vi "FTT Init Display.vi"(8 "error in (no error)":errorcluster caption="错误输入（无错误）", 11 "Cluster 2":T4) -> (0 "error out":errorcluster caption="错误输出", 3 "Cluster out":T4)   [LabVIEW 2014]
uses:
  <vilib>/picture/picture.llb/imagedata.ctl
  Type'def/CN Config Ctr.ctl
  Type'def/CN image Ctr.ctl
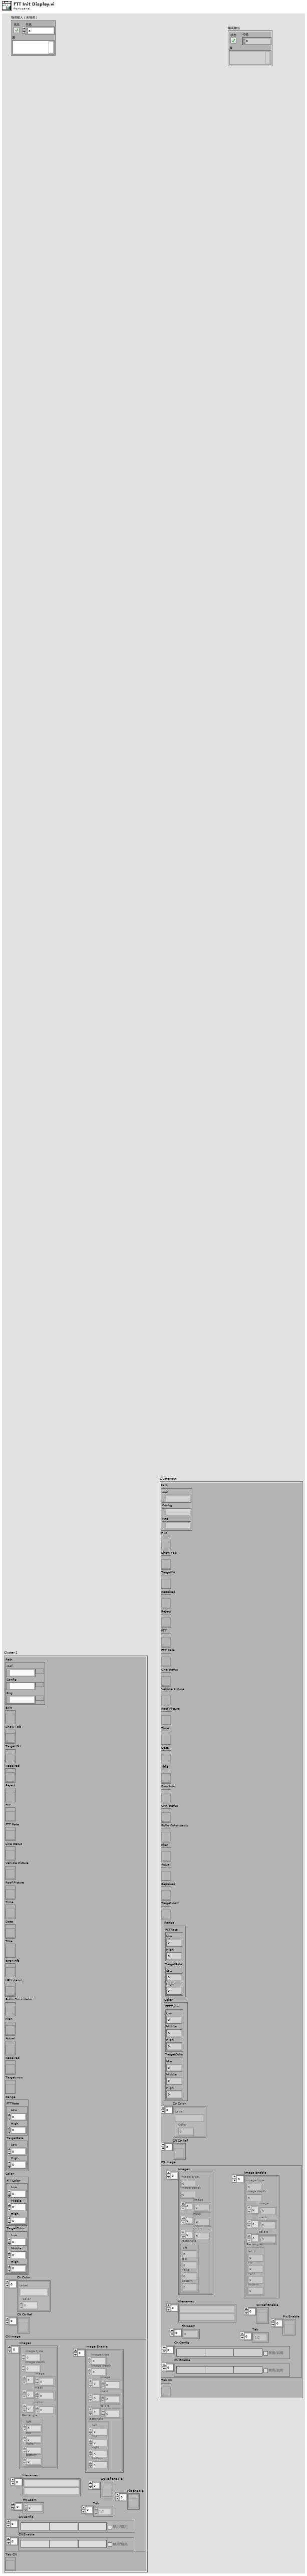
[diagram p1: front panel]
types:
  T1 = typedef "CN image Ctr.ctl" = cluster{"Images":T2[], "filenames":string[], "Fit Zoom":dbl[], "CN Config":T3[], "CN Enable":T3[], "image Enable":T2[], "CN Ref Enable":refnum<vi>[], "Tab ":enum32{"1/2", "1/3", "1/4", "1/5", "2/5", "3/5"}[], "Pic Enable":refnum<vi>[]}
  T2 = typedef "imagedata.ctl" = cluster{"image type":i32, "image depth":i32, "image":u8[], "mask":u8[], "colors":u32[], "Rectangle":cluster{"left":i16, "top":i16, "right":i16, "bottom":i16}}
  T3 = typedef "CN Config Ctr.ctl" = cluster{"Model":string, "Pic_Name":string, "CarName":string, "En/Disable":bool}
  T4 = cluster{"Path":cluster{"roof":path, "Config":path, "Png":path}, "Exit":refnum<vi>, "Show Tab":refnum<vi>, "Target(%)":refnum<vi>, "Repaired":refnum<vi>, "Reject":refnum<vi>, "FTT":refnum<vi>, "FTT Rate":refnum<vi>, "Line status":refnum<vi>, "Vehicle Picture":refnum<vi>, "Roof Picture":refnum<vi>, "Time":refnum<vi>, "Date":refnum<vi>, "Title":refnum<vi>, "Error Info":refnum<vi>, "UPH status":refnum<vi>, "Rollo Color status":refnum<vi>, "Plan":refnum<vi>, "Actual":refnum<vi>, "Repaired":refnum<vi>, "Target now":refnum<vi>, "Range":cluster{"FTTRate":cluster{"Low":u32, "High":u32}, "TargetRate":cluster{"Low":u32, "High":u32}}, "Color":cluster{"FTTColor":cluster{"Low":u32, "Middle":u32, "High":u32}, "TargetColor":cluster{"Low":u32, "Middle":u32, "High":u32}}, "Ctr Color":cluster{"Label":string, "Color":u32}[], "CN Ctr Ref":refnum<vi>[], "CN image":T1, "Tab CN":refnum<vi>}
  T5 = enum8{"Enabled", "Disabled", "Disabled and Grayed Out"}
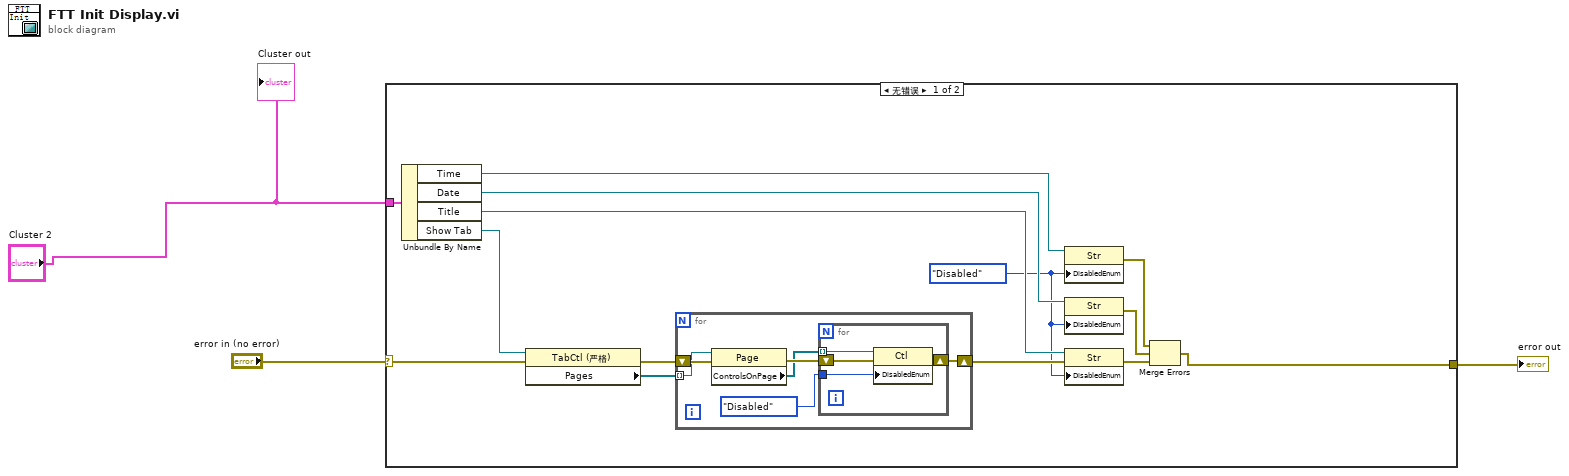
[diagram p0: block diagram]
diagram:
  n1 = case shown="无错误" "error in (no error)" {
    selector: "error in (no error)" -> [w13 w28]
    tunnel: "Cluster 2" -> [w17 _]
    tunnel: [w4 w28] -> w2
    frame No Error {
      w5 = T5."Disabled" ("禁用")
      n2 = Unbundle By Name(w17) -> ("Time"=w9:refnum<vi>, "Date"=w10:refnum<vi>, "Title"=w11:refnum<vi>, "Show Tab"=w16:refnum<vi>)
      n3 = property class="TabCtl (严格)"(reference=w16, error in=w13) -> (error out=w15:errorcluster, "Pages"=w14:refnum<vi>[])  [unwired: 1 out]
      n4 = for {
        tunnel: w14 -> [w22] mode=indexing
        shift-right: [w18] -> w12
        shift-left: w15 -> [w23]
        n5 = property class="Page"(reference=w22, error in=w23) -> (error out=w21:errorcluster, "ControlsOnPage"=w20:refnum<vi>[])  [unwired: 1 out]
        n6 = for {
          tunnel: w20 -> [w26] mode=indexing
          tunnel: T5."Disabled" ("禁用") -> [w25]
          shift-right: [w24] -> w18
          shift-left: w21 -> [w27]
          n7 = property class="Ctl"(reference=w26, error in=w27, "DisabledEnum"=w25) -> (error out=w24:errorcluster)  [unwired: 1 out]
        }
      }
      n8 = property class="Str"(reference=w9, "DisabledEnum"=w5) -> (error out=w6:errorcluster)  [unwired: 1 in, 1 out]
      n9 = property class="Str"(reference=w10, "DisabledEnum"=w5) -> (error out=w7:errorcluster)  [unwired: 1 in, 1 out]
      n10 = property class="Str"(reference=w11, error in=w12, "DisabledEnum"=w5) -> (error out=w8:errorcluster)  [unwired: 1 out]
      n11 = Merge Errors(w6, w7, w8) -> (w4:errorcluster)
    }
    frame Error {
    }
  }
  "error out" <- w2
  "Cluster out" <- "Cluster 2"
